vi "VWflipperScalar.vi"(4 "Probe Orientation":u16(ring)=90 items=["Horizontal"=0, "Diagonal"=45, "Vertical"=90, "User Defined"=999], 6 "Probe Type":u16(ring)=5 items=["5-Hole Probe"=5, "OmniProbe"=12], 7 "Theta Degree":dbl, 8 "Probe w m/s":dbl, 9 "Probe v m/s":dbl, 10 "Probe u  m/s":dbl, 11 "VMagn m/s":dbl) -> (3 "VmagUVWCone":dbl[](array[numeric]))   [LabVIEW 2016]
uses:
  <vilib>/Analysis/coordinate.llb/Euler Rotation Order.ctl
  <vilib>/Analysis/coordinate.llb/3D Cartesian Coordinate Rotation (Euler) (Scalar).vi
  <vilib>/Analysis/NI_AALPro.lvlib
panel:
  in  "User-Defined Euler Angles":cluster{"phi":dbl, "theta":dbl, "psi":dbl}
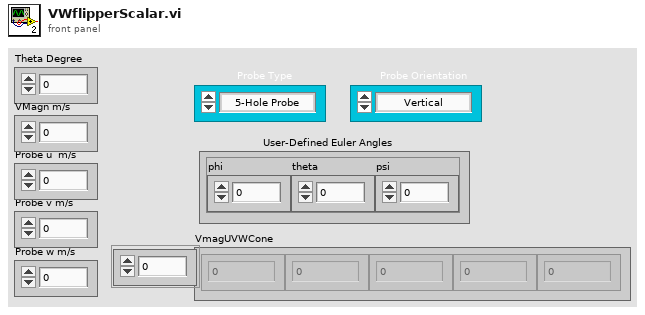
[diagram p1: front panel]
types:
  T1 = typedef "NI_AALPro.lvlib/Euler Rotation Order.ctl" = u16
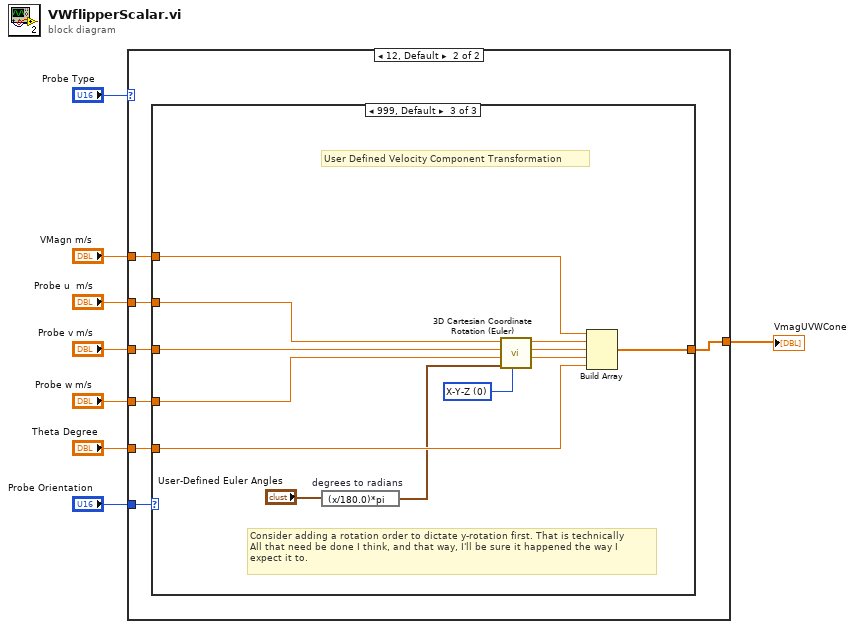
[diagram p0: block diagram]
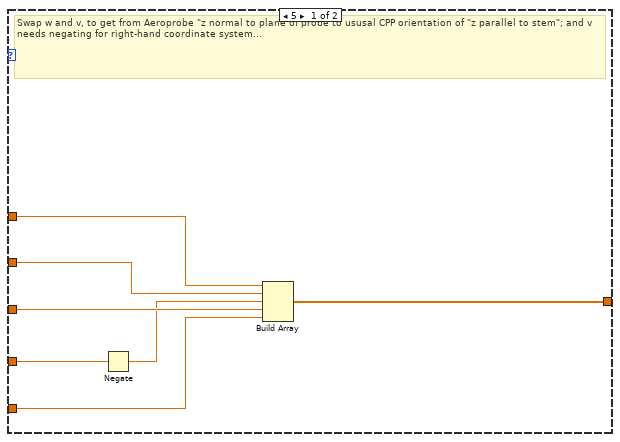
[diagram p2: hidden frame]
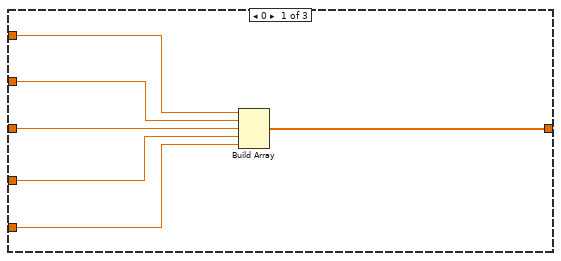
[diagram p3: hidden frame]
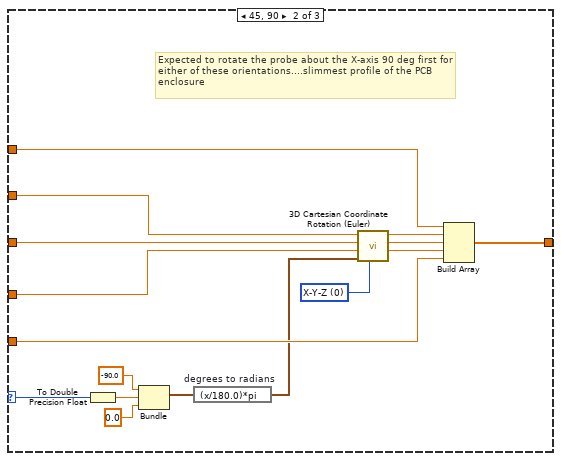
[diagram p4: hidden frame]
diagram:
  n1 = case shown="12, Default" "Probe Type" {
    tunnel: "Theta Degree" -> [w15 w22]
    tunnel: "Probe w m/s" -> [w14 w17]
    tunnel: "Probe v m/s" -> [w13 w18]
    tunnel: "Probe u  m/s" -> [w11 w21]
    tunnel: "VMagn m/s" -> [w10 w20]
    tunnel: [w9 w19] -> w6
    tunnel: "Probe Orientation" -> [_ w16]
    frame 5 {
      # "Swap w and v, to get from Aeroprobe \"z normal to plane of probe to ususal CPP orientation of \"z parallel to stem\"; and v needs negating for right-hand coordinate system..."
      n2 = Negate(x=w14) -> (-x=w12:dbl)
      n3 = Build Array(w10, w11, w12, w13, w15) -> (w9:dbl[])
    }
    frame 12, Default {
      n4 = case shown="999, Default" w16 {
        selector: w16 -> [_ w38 _]
        tunnel: w22 -> [w28 w44 w56]
        tunnel: w21 -> [w27 w40 w52]
        tunnel: w20 -> [w26 w43 w55]
        tunnel: [w25 w42 w54] -> w19
        tunnel: w18 -> [w24 w41 w53]
        tunnel: w17 -> [w23 w39 w51]
        frame 0 {
          n5 = Build Array(w26, w27, w24, w23, w28) -> (w25:dbl[])
        }
        frame 45, 90 {
          w34 = T1 0 items=["X-Y-Z", "X-Z-Y", "Y-X-Z", "Y-Z-X", "Z-X-Y", "Z-Y-X", "X-Y-X", "X-Z-X", "Y-X-Y", "Y-Z-Y", "Z-X-Z", "Z-Y-Z"] ("rotation order")
          # "Expected to rotate the probe about the X-axis 90 deg first for either of these orientations....slimmest profile of the PCB enclosure"
          n6 = To Double Precision Float(number=w38) -> (double precision float=w31:dbl)
          n7 = Bundle("phi"=-90.0, w31, "theta"=0.0) -> (w30:cluster{"phi":dbl, dbl, "theta":dbl})  [unwired: 1 in]
          n8 = expression code="(x/180.0)*pi" "degrees to radians"(w30) -> (w29:cluster{"phi":dbl, dbl, "theta":dbl})
          n9 = call-poly <vilib>:"3D Cartesian Coordinate Rotation (Euler).vi"("rotation order"=w34, "Euler Angles"=w29, "z"=w39, "y"=w41, "x"=w40) -> ("z out"=w35:dbl, "y out"=w36:dbl, "x out"=w37:dbl)  [unwired: 3 in, 1 out]
          n10 = Build Array(w43, w37, w36, w35, w44) -> (w42:dbl[])
        }
        frame 999, Default {
          w47 = T1 0 items=["X-Y-Z", "X-Z-Y", "Y-X-Z", "Y-Z-X", "Z-X-Y", "Z-Y-X", "X-Y-X", "X-Z-X", "Y-X-Y", "Y-Z-Y", "Z-X-Z", "Z-Y-Z"] ("rotation order")
          # "User Defined Velocity Component Transformation"
          # "Consider adding a rotation order to dictate y-rotation first. That is technically\nAll that need be done I think, and that way, I'll be sure it happened the way I\nexpect it to."
          n11 = expression code="(x/180.0)*pi" "degrees to radians"("User-Defined Euler Angles") -> (w45:cluster{"phi":dbl, "theta":dbl, "psi":dbl})
          n12 = call-poly <vilib>:"3D Cartesian Coordinate Rotation (Euler).vi"("rotation order"=w47, "Euler Angles"=w45, "z"=w51, "y"=w53, "x"=w52) -> ("z out"=w48:dbl, "y out"=w49:dbl, "x out"=w50:dbl)  [unwired: 3 in, 1 out]
          n13 = Build Array(w55, w50, w49, w48, w56) -> (w54:dbl[])
        }
      }
    }
  }
  "VmagUVWCone" <- w6
